vi "rszvl Marker Search.vi"(7 "Search (Max)":i32(ring) items=["Max", "Min", "Right Peak", "Left Peak", "Next Peak"], 8 "error in (no error)":errorcluster, 9 "Marker (1)":i32=1, 10 "Channel (1)":i32=1, 11 "VISA resource name":refnum<visa-resource-name>) -> (0 "error out":errorcluster, 3 "VISA resource name out":refnum<visa-resource-name>)   [LabVIEW 2014]
doc: "This VI searches with the active marker for specific points on the trace.\n\nNote(s):\n\nThe marker must be created before using CALCulate<Ch/Tr>:MARKer<Mk>[:STATe] ON.\n\nAttribute(s):\nRSZVL_ATTR_NWA_MARKER_SEARCH_MODE\n\nRemote-control command(s):\nCALCulate<Ch/Tr>:MARKer<Mk>:FUNCtion:EXECute MAXimum | MINimum | NPEak | RPEak | LPEak"
uses:
  Instance           1 27Saved   rszvl Marker Search .vi
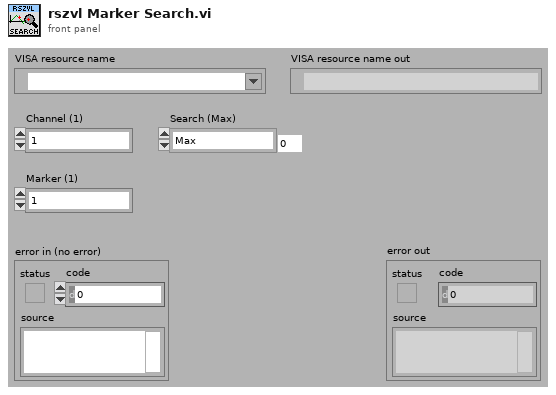
[diagram p1: front panel]
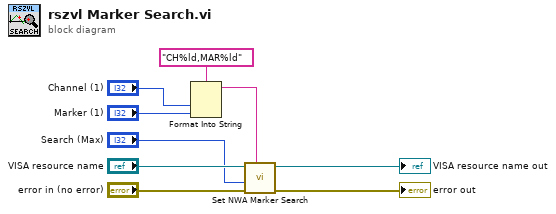
[diagram p0: block diagram]
diagram:
  n1 = Format Into String(format string="CH%ld,MAR%ld", "Channel (1)", "Marker (1)") -> (resulting string=w8:string)  [unwired: 2 in, 1 out]
  n2 = call "Set NWA Marker Search"("Repeated Capabilities"=w8, "error in (no error)"="error in (no error)", "NWA Marker Search (0 - MARK_SEARCH_MAX)"="Search (Max)", "instrument handle"="VISA resource name") -> ("error out"=→"error out":errorcluster, "instrument handle out"=→"VISA resource name out":refnum<visa-resource-name>)  [unwired: 6 in]
